vi "进账写入数据库.vi"(10 "输出簇":T1) -> ()   [LabVIEW 2010]
panel:
  in  "簇":cluster{"字符串":string, "下拉列表":u16}
  in  "error in (no error)":errorcluster caption="错误输入（无错误）"
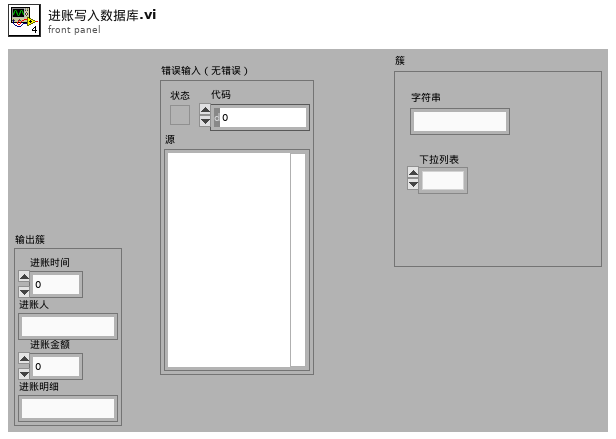
[diagram p1: front panel]
types:
  T1 = cluster{"进账时间":u64, "进账人":string, "进账金额":dbl, "进账明细":string}
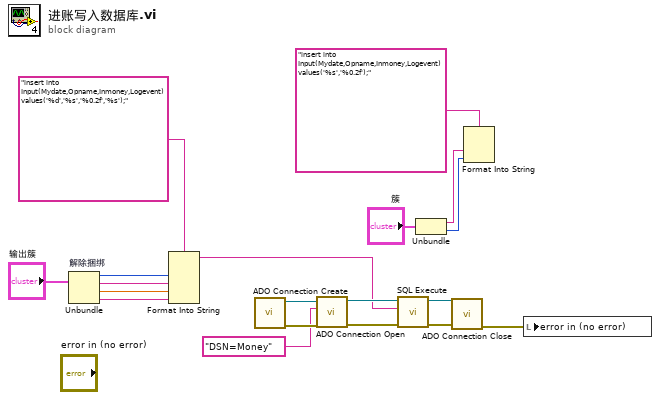
[diagram p0: block diagram]
diagram:
  n1 = Unbundle "解除捆绑"("输出簇") -> ("进账时间"=w5:u64, "进账人"=w10:string, "进账金额"=w9:dbl, "进账明细"=w8:string)
  n2 = Format Into String(format string="insert into Input(Mydate,Opname,Inmoney,Logevent) values('%d','%s','%0.2f','%s');", w5, w10, w9, w8) -> (resulting string=w6:string)  [unwired: 2 in, 1 out]
  n3 = call "ADO Connection Create.vi"() -> ("error out"=w19:errorcluster, "ADODB._Connection Out"=w18:refnum<k7>)  [unwired: 10 in]
  n4 = call "ADO Connection Open.vi"("error in (no error)"=w19, "ConnectionString"="DSN=Money", "ADODB._Connection In"=w18) -> ("error out"=w14:errorcluster, "ADODB._Connection Out"=w15:refnum<k7>)  [unwired: 7 in]
  n5 = call "SQL Execute.vi"("error in (no error)"=w14, "Command Text"=w6, "ADODB._Connection In"=w15) -> ("error out"=w12:errorcluster, "ADODB._Connection Out"=w13:refnum<k7>)  [unwired: 5 in, 2 out]
  n6 = Unbundle("簇") -> ("字符串"=w3:string, "下拉列表"=w2:u16)
  n7 = call "ADO Connection Close.vi"("error in (no error)"=w12, "ADODB._Connection In"=w13) -> ("error out"=w16:errorcluster)  [unwired: 8 in, 1 out]
  n8 = Format Into String(format string="insert into Input(Mydate,Opname,Inmoney,Logevent) values('%s','%0.2f');", w3, w2) -> ()  [unwired: 2 in, 2 out]
  n9 = local write "error in (no error)"(w16) -> ()
